vi "(SubVI)_Average_MultiSite_mising_frm_handling.vi"(8 "Size MAF":dbl, 9 "Current Index":dbl, 10 "Frm# Array":dbl[][](array[numeric]), 11 "Dpp Array":dbl[][](array[numeric])) -> (3 "Average":dbl[](array[numeric]))   [LabVIEW 2019]
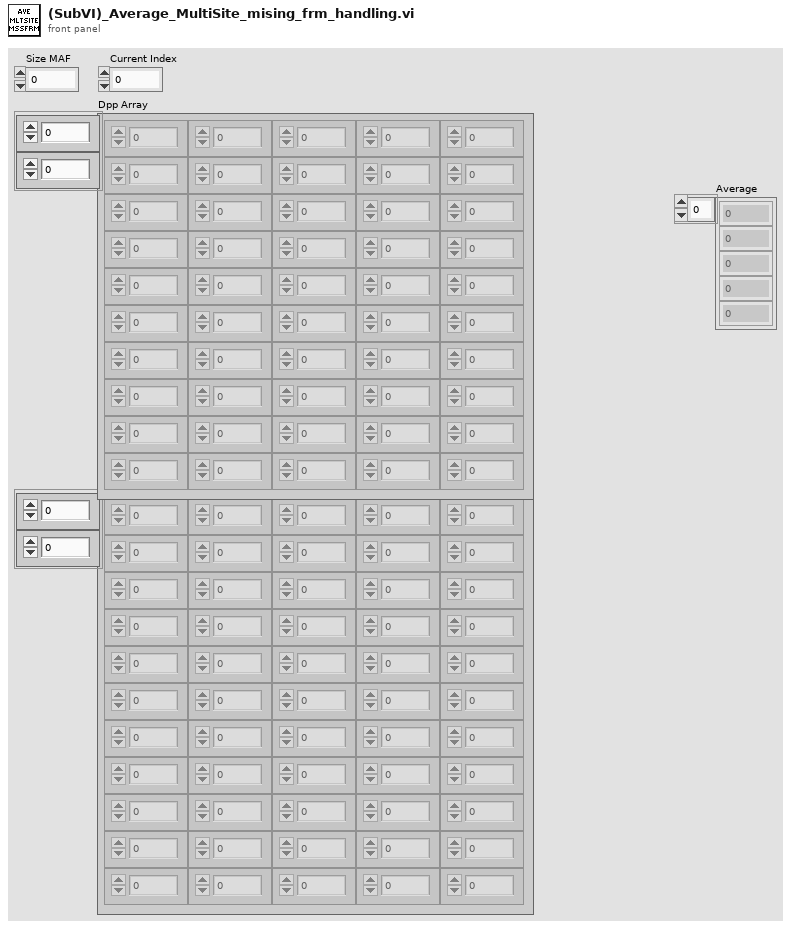
[diagram p1: front panel]
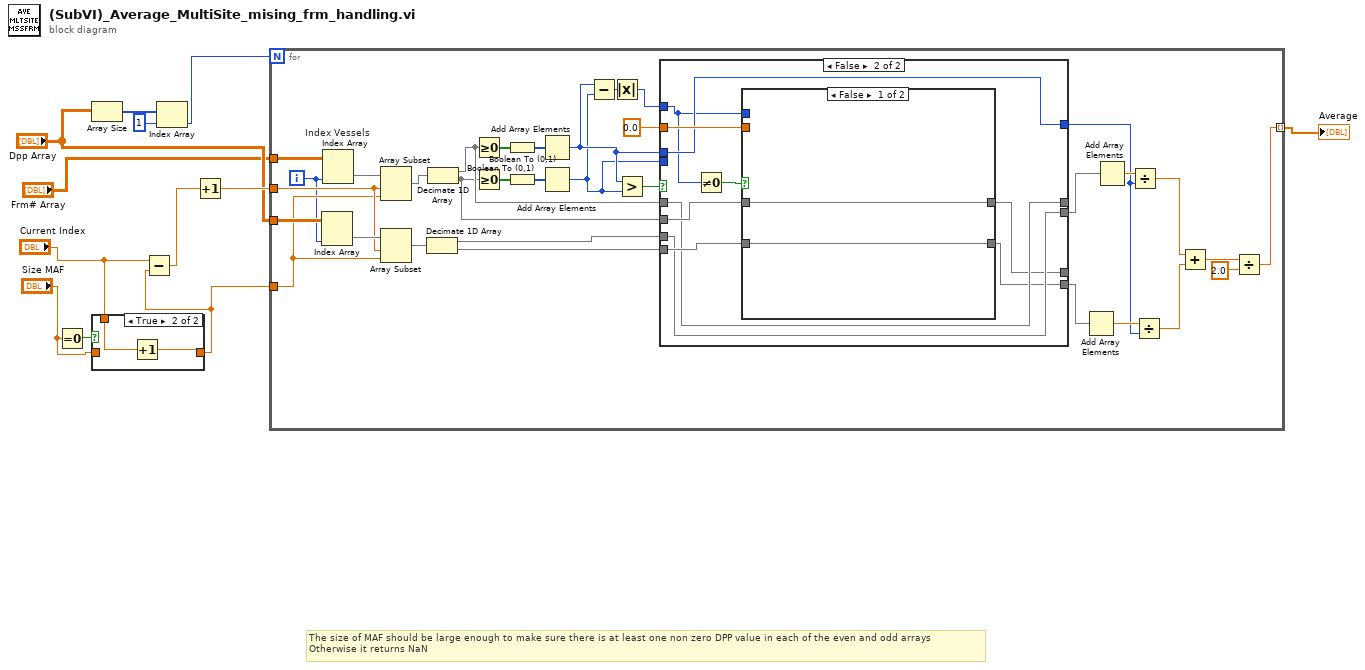
[diagram p0: block diagram]
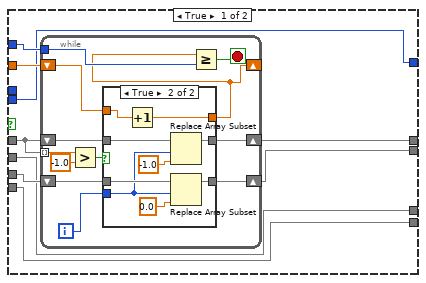
[diagram p3: hidden frame]
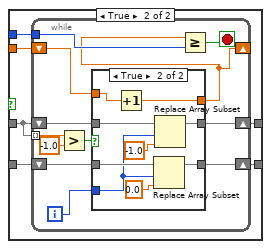
[diagram p5: hidden frame]
diagram:
  # "The size of MAF should be large enough to make sure there is at least one non zero DPP value in each of the even and odd arrays\nOtherwise it returns NaN"
  n1 = Equal To 0?(x="Size MAF") -> (x = 0?=w4:bool)
  n2 = Array Size(array="Dpp Array") -> (size(s)=w12:i32[])
  n3 = case shown="True" w4 {
    tunnel: "Size MAF" -> [w13 _]
    tunnel: [w13 w14] -> w2
    tunnel: "Current Index" -> [_ w15]
    frame False {
    }
    frame True {
      n4 = Increment(x=w15) -> (x+1=w14:dbl)
    }
  }
  n5 = Subtract(x="Current Index", y=w2) -> (x-y=w8:dbl)
  n6 = Index Array(array=w12, index=1) -> (element=w10:i32)
  n7 = Increment(x=w8) -> (x+1=w7:dbl)
  n8 = for {
    N: w10 -> [_]
    tunnel: "Dpp Array" -> [w48]
    tunnel: "Frm# Array" -> [w47]
    tunnel: [w35] -> w9 mode=indexing
    tunnel: w2 -> [w24]
    tunnel: w7 -> [w25]
    i -> [w16]
    n9 = Index Array(array=w48, index (col)=w16) -> (element=w27:dbl[])  [unwired: 1 in]
    n10 = Index Array "Index Vessels"(array=w47, index (col)=w16) -> (element=w46:dbl[])  [unwired: 1 in]
    n11 = Array Subset(array=w46, index=w25, length=w24) -> (w17:dbl[])
    n12 = Array Subset(array=w27, index=w25, length=w24) -> (w26:dbl[])
    n13 = Decimate 1D Array(w26) -> (w31:dbl[], w23:dbl[])
    n14 = Decimate 1D Array(w17) -> (w28:dbl[], w18:dbl[])
    n15 = Greater Or Equal To 0?(x=w28) -> (x >= 0?=w45:bool[])
    n16 = Greater Or Equal To 0?(x=w18) -> (x >= 0?=w44:bool[])
    n17 = Boolean To (0,1)(Boolean=w45) -> (0, 1=w43:i16[])
    n18 = Boolean To (0,1)(Boolean=w44) -> (0, 1=w42:i16[])
    n19 = Add Array Elements(numeric array=w43) -> (sum=w29:i16)
    n20 = Add Array Elements(numeric array=w42) -> (sum=w22:i16)
    n21 = Subtract(x=w29, y=w22) -> (x-y=w34:i16)
    n22 = Absolute Value(x=w34) -> (abs(x)=w30:i16)
    n23 = Greater?(x=w29, y=w22) -> (0:w32:bool)
    n24 = case shown="False" w32 {
      tunnel: w31 -> [w55 w87]
      tunnel: 0.0 -> [w57 w91]
      tunnel: w30 -> [w56 w82]
      tunnel: w29 -> [_ w84]
      tunnel: w28 -> [w54 w88]
      tunnel: w18 -> [w52 w90]
      tunnel: w23 -> [w50 w89]
      tunnel: [w53 w88] -> _
      tunnel: [w52 w86] -> _
      tunnel: [w51 w87] -> w20
      tunnel: [w50 w85] -> w19
      tunnel: [w49 w84] -> w21
      tunnel: w22 -> [w49 _]
      frame True {
        n25 = while {
          tunnel: w56 -> [w68]
          tunnel: w54 -> [w67] mode=indexing
          shift-right: [w61] -> w53
          shift-left: w54 -> [w64]
          shift-right: [w60] -> w51
          shift-left: w55 -> [w62]
          shift-right: [w58] -> _
          shift-left: w57 -> [w59]
          i -> [w63]
          stop <- w69 stop-if-true
          n26 = Greater?(x=w67, y=-1.0) -> (0:w66:bool)
          n27 = case shown="True" w66 {
            tunnel: w64 -> [w72 w81]
            tunnel: w63 -> [_ w77]
            tunnel: w62 -> [w71 w78]
            tunnel: [w72 w79] -> w61
            tunnel: [w71 w75] -> w60
            tunnel: w59 -> [w70 w74]
            tunnel: [w70 w73] -> w58
            frame False {
            }
            frame True {
              n28 = Increment(x=w74) -> (x+1=w73:dbl)
              n29 = Replace Array Subset(array=w81, new element=-1.0 ("new element/subarray"), index=w77) -> (w79:dbl[])
              n30 = Replace Array Subset(array=w78, new element=0.0 ("new element/subarray"), index=w77) -> (w75:dbl[])
            }
          }
          n31 = Greater Or Equal?(x=w58, y=w68) -> (x >= y?=w69:bool)
        }
      }
      frame False {
        n32 = Not Equal To 0?(x=w82) -> (x != 0?=w83:bool)
        n33 = case shown="False" w83 {
          tunnel: w91 -> [_ w99]
          tunnel: w82 -> [_ w98]
          tunnel: w90 -> [w93 w97]
          tunnel: w89 -> [w92 w96]
          tunnel: [w93 w95] -> w86
          tunnel: [w92 w94] -> w85
          frame False {
          }
          frame True {
            n34 = while {
              tunnel: w98 -> [w110]
              tunnel: w97 -> [w109] mode=indexing
              shift-right: [w103] -> w95
              shift-left: w97 -> [w106]
              shift-right: [w102] -> w94
              shift-left: w96 -> [w104]
              shift-right: [w100] -> _
              shift-left: w99 -> [w101]
              i -> [w105]
              stop <- w111 stop-if-true
              n35 = Greater?(x=w109, y=-1.0) -> (0:w108:bool)
              n36 = case shown="True" w108 {
                tunnel: w106 -> [w114 w123]
                tunnel: w105 -> [_ w119]
                tunnel: w104 -> [w113 w120]
                tunnel: [w114 w121] -> w103
                tunnel: [w113 w117] -> w102
                tunnel: w101 -> [w112 w116]
                tunnel: [w112 w115] -> w100
                frame False {
                }
                frame True {
                  n37 = Increment(x=w116) -> (x+1=w115:dbl)
                  n38 = Replace Array Subset(array=w120, new element=0.0 ("new element/subarray"), index=w119) -> (w117:dbl[])
                  n39 = Replace Array Subset(array=w123, new element=-1.0 ("new element/subarray"), index=w119) -> (w121:dbl[])
                }
              }
              n40 = Greater Or Equal?(x=w100, y=w110) -> (x >= y?=w111:bool)
            }
          }
        }
      }
    }
    n41 = Add Array Elements(numeric array=w19) -> (sum=w41:dbl)
    n42 = Add Array Elements(numeric array=w20) -> (sum=w40:dbl)
    n43 = Divide(x=w40, y=w21) -> (x/y=w39:dbl)
    n44 = Divide(x=w41, y=w21) -> (x/y=w38:dbl)
    n45 = Add(x=w39, y=w38) -> (x+y=w37:dbl)
    n46 = Divide(x=w37, y=2.0) -> (x/y=w35:dbl)
  }
  "Average" <- w9
